vi "Multiply Rational Polynomials (CDB).vi"(4 "threshold type":T1 items=["Absolute Value", "Relative Value"], 6 "threshold":dbl, 8 "Denominator 2":cdb[](array[numeric]) format="%#.2g", 9 "Numerator 2":cdb[](array[numeric]) format="%#.2g", 10 "Denominator 1":cdb[](array[numeric]) format="%#.2g", 11 "Numerator 1":cdb[](array[numeric]) format="%#.2g") -> (0 "error":i32, 2 "Denominator Out":cdb[](array[numeric]) format="%#.2g", 3 "Numerator Out":cdb[](array[numeric]) format="%#.2g")   [LabVIEW 2017, in "NI_AALPro.lvlib"]
doc: "Multiplies rational polynomial G1 by rational polynomial G2. The data types you wire to the <B>Numerator 1</B>, <B>Denominator 1</B>, <B>Numerator 2</B>, and <B>Denominator 2</B> inputs determine the polymorphic instance to use."
uses:
  NI_AALPro.lvlib
  Remove Zero Threshold Type.ctl
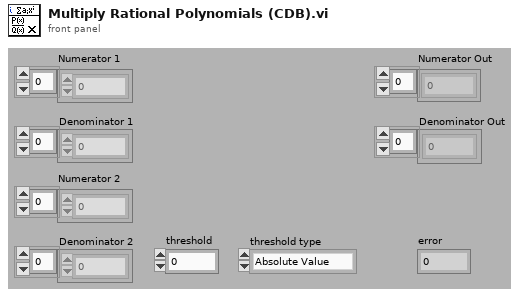
[diagram p1: front panel]
types:
  T1 = typedef "NI_AALPro.lvlib/Remove Zero Threshold Type.ctl" = u16
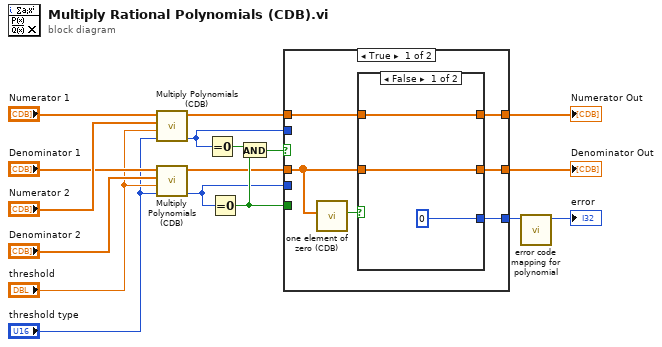
[diagram p0: block diagram]
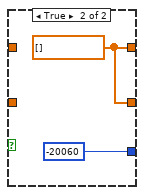
[diagram p2: hidden frame]
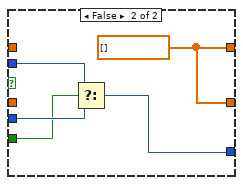
[diagram p3: hidden frame]
diagram:
  n1 = call "Multiply Polynomials (CDB).vi"("threshold type"="threshold type", "threshold"="threshold", "Q(x)"="Numerator 2", "P(x)"="Numerator 1") -> ("error"=w7:i32, "P(x)*Q(x)"=w8:cdb[])  [unwired: 6 in]
  n2 = call "Multiply Polynomials (CDB).vi"("threshold type"="threshold type", "threshold"="threshold", "Q(x)"="Denominator 2", "P(x)"="Denominator 1") -> ("error"=w3:i32, "P(x)*Q(x)"=w4:cdb[])  [unwired: 6 in]
  n3 = Equal To 0?(x=w7) -> (x = 0?=w13:bool)
  n4 = Equal To 0?(x=w3) -> (x = 0?=w11:bool)
  n5 = And(x=w13, y=w11) -> (x .and. y?=w12:bool)
  n6 = case shown="True" w12 {
    tunnel: w8 -> [w23 _]
    tunnel: w4 -> [w19 _]
    tunnel: [w22 w33] -> w17
    tunnel: [w21 w33] -> w16
    tunnel: [w18 w30] -> w15
    tunnel: w7 -> [_ w32]
    tunnel: w3 -> [_ w31]
    tunnel: w11 -> [_ w29]
    frame True {
      n7 = call "one element of zero (CDB).vi"("Array in"=w19) -> ("equal [0]?"=w20:bool)  [unwired: 10 in]
      n8 = case shown="False" w20 {
        tunnel: w23 -> [w26 _]
        tunnel: [w26 w28] -> w22
        tunnel: w19 -> [w25 _]
        tunnel: [w25 w28] -> w21
        tunnel: [0 -20060 ("divide by zero")] -> w18
        frame False {
        }
        frame True {
          w28 = cdb[] [] ("CDB")
        }
      }
    }
    frame False {
      w33 = cdb[] [] ("CDB")
      n9 = Select(t=w32, s=w29, f=w31) -> (s? t:f=w30:i32)
    }
  }
  "Numerator Out" <- w17
  "Denominator Out" <- w16
  n10 = call "error code mapping for polynomial.vi"("error in"=w15) -> ("error out"=→"error":i32)  [unwired: 10 in]
